vi "Creators All Created Queues.vi"(9 "Priority?":bool, 10 "Msg Strategy":refnum<class "Msg Strategy.lvclass">, 11 "Base Event in":refnum<class "Base Event.lvclass">) -> (3 "Base Event out":refnum<class "Base Event.lvclass">)   [LabVIEW 2021, in "jettl.lvlib" / "Base Event.lvlib" / "Base Event.lvclass"]
uses:
  Base Event.lvclass
  Base Event.lvclass/Base Event.ctl
  Msg Strategy/Msg Strategy.lvclass
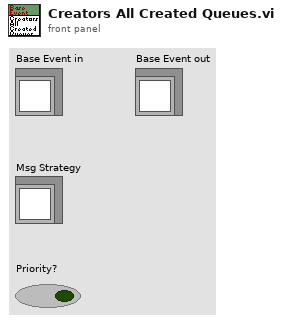
[diagram p1: front panel]
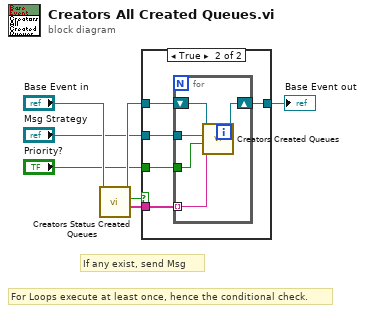
[diagram p0: block diagram]
diagram:
  # "For Loops execute at least once, hence the conditional check."
  # "If any exist, send Msg"
  n1 = call-dynamic "Creators Status Created Queues.vi"("Base Event in"="Base Event in") -> ("Created Queue Aliases"=w1:string[], "Created Queue Exist?"=w2:bool, "Base Event out"=w7:refnum<class "Base Event.lvclass">)  [unwired: 7 in, 1 out]
  n2 = case shown="True" w2 {
    tunnel: [w8 w13] -> w3
    tunnel: w7 -> [w8 w12]
    tunnel: w1 -> [_ w11]
    tunnel: "Msg Strategy" -> [_ w10]
    tunnel: "Priority?" -> [_ w9]
    frame False {
    }
    frame True {
      n3 = for {
        tunnel: w11 -> [w14] mode=indexing
        shift-right: [w17] -> w13
        shift-left: w12 -> [w18]
        tunnel: w10 -> [w16]
        tunnel: w9 -> [w15]
        n4 = call-dynamic "Creators Created Queues.vi"("Created Queue Alias"=w14, "Priority?"=w15, "Msg Strategy"=w16, "Base Event in"=w18) -> ("Base Event out"=w17:refnum<class "Base Event.lvclass">)  [unwired: 7 in]
      }
    }
  }
  "Base Event out" <- w3
